vi "Format_Readout_Data.vi"(7 "Raw Spec Const 2":i32[](array[numeric]), 8 "Channel Name":string, 10 "Raw Spec Const":i32[](array[numeric]), 11 "Data packet":u8[](array[numeric])) -> (0 "Channel names":string[](array[string]), 1 "Raw Spectrum":i32[](array[numeric]), 2 "Total Integral":i32[](array[numeric]), 3 "Tail Integral":i32[](array[numeric]), 5 "Raw Spectrum 2":i32[](array[numeric]))   [LabVIEW 2015]
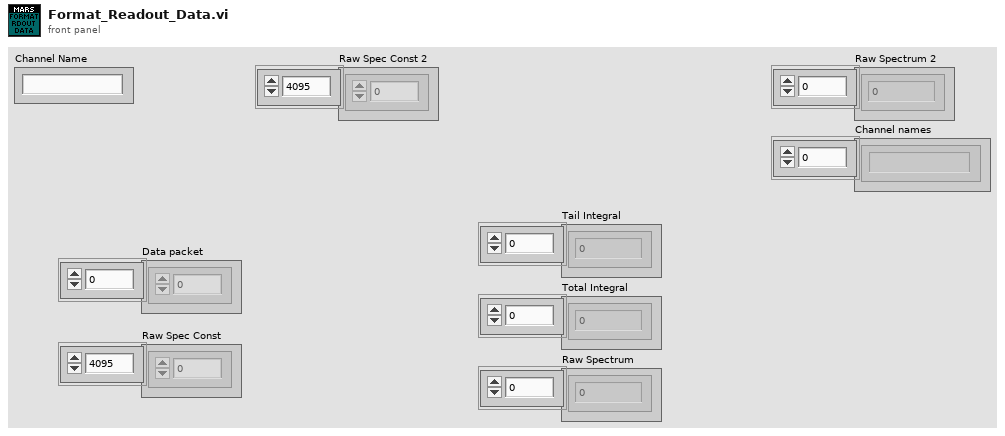
[diagram p1: front panel]
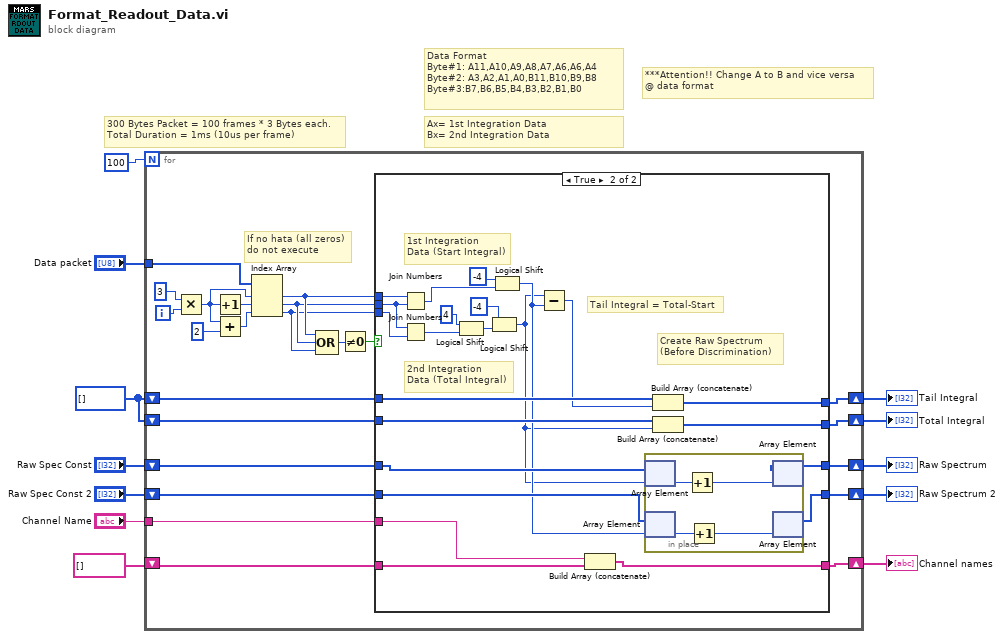
[diagram p0: block diagram]
diagram:
  w4 = u16[] []
  # "***Attention!! Change A to B and vice versa\n@ data format"
  # "300 Bytes Packet = 100 frames * 3 Bytes each.\nTotal Duration = 1ms (10us per frame)"
  # "Ax= 1st Integration Data\nBx= 2nd Integration Data"
  # "Data Format\nByte#1: A11,A10,A9,A8,A7,A6,A6,A4\nByte#2: A3,A2,A1,A0,B11,B10,B9,B8\nByte#3:B7,B6,B5,B4,B3,B2,B1,B0"
  n1 = for {
    N: 100 -> [_]
    tunnel: "Data packet" -> [w33]
    shift-right: [w22] -> w7
    shift-left: w4 -> [w23]
    shift-right: [w20] -> w10
    shift-left: w4 -> [w21]
    shift-right: [w18] -> w11
    shift-left: "Raw Spec Const" -> [w19]
    shift-right: [w16] -> w5
    shift-left: "Raw Spec Const 2" -> [w17]
    shift-right: [w14] -> w1
    shift-left: string[] [] -> [w15]
    tunnel: "Channel Name" -> [w13]
    i -> [w35]
    # "If no hata (all zeros)\ndo not execute"
    n2 = Multiply(x=3, y=w35) -> (x*y=w31:i32)
    n3 = Increment(x=w31) -> (x+1=w32:i32)
    n4 = Add(x=w31, y=2 ("x")) -> (x+y=w29:i32)
    n5 = Index Array(array=w33, index #1=w31, index #2=w32, index #3=w29) -> (element #1=w26:u8, element #2=w25:u8, element #3=w24:u8)
    n6 = Compound Arithmetic op=OR(w26, w25, w24) -> (w28:u8)
    n7 = Not Equal To 0?(x=w28) -> (x != 0?=w27:bool)
    n8 = case shown="True" w27 {
      tunnel: w26 -> [_ w61]
      tunnel: w25 -> [_ w56]
      tunnel: w24 -> [_ w55]
      tunnel: w23 -> [w40 w54]
      tunnel: [w40 w53] -> w22
      tunnel: w21 -> [w39 w52]
      tunnel: [w39 w51] -> w20
      tunnel: w19 -> [w38 w50]
      tunnel: [w38 w49] -> w18
      tunnel: w17 -> [w37 w48]
      tunnel: [w37 w47] -> w16
      tunnel: w15 -> [w36 w44]
      tunnel: [w36 w43] -> w14
      tunnel: w13 -> [_ w42]
      frame False {
      }
      frame True {
        # "Create Raw Spectrum\n(Before Discrimination)"
        # "Tail Integral = Total-Start"
        # "2nd Integration\nData (Total Integral)"
        # "1st Integration\nData (Start Integral)"
        n9 = Join Numbers(hi=w61, lo=w56) -> ((hi.lo)=w62:u16)
        n10 = Join Numbers(hi=w56, lo=w55) -> ((hi.lo)=w58:u16)
        n11 = Logical Shift(y=i8 4, x=w58) -> (x << y=w60:u16)
        n12 = Logical Shift(y=i8 -4, x=w60) -> (x << y=w41:u16)
        n13 = Logical Shift(y=i8 -4, x=w62) -> (x << y=w45:u16)
        n14 = Subtract(x=w41, y=w45) -> (x-y=w46:u16)
        n15 = Build Array (concatenate)(w42, w44) -> (w43:string[])
        n16 = in-place {
          n17 = in-place-array #1(w50, w41) -> (w67:i32)
          n18 = in-place-array #2(w48, w45) -> (w65:i32)
          n19 = Increment(x=w67) -> (x+1=w66:i32)
          n20 = Increment(x=w65) -> (x+1=w64:i32)
          n21 = in-place-array #1(w66) -> (w49:i32[])  [unwired: 1 out]
          n22 = in-place-array #2(w64) -> (w47:i32[])  [unwired: 1 out]
        }
        n23 = Build Array (concatenate)(w54, w46) -> (w53:u16[])
        n24 = Build Array (concatenate)(w52, w41) -> (w51:u16[])
      }
    }
  }
  "Total Integral" <- w10
  "Tail Integral" <- w7
  "Raw Spectrum" <- w11
  "Raw Spectrum 2" <- w5
  "Channel names" <- w1
